vi "WriteRegisterArray.vi"(6 "Pause":u32, 7 "Mode":enum16{"Normal", "Config"}(ring), 8 "WriteSize":enum16{"1", "2", "4"}(ring), 9 "SclkDivider":u32=2, 10 "NumReg":i16, 11 "Register  Values":cluster{"Address":u8, "Value":u32}[](array[cluster])=[{"Address"=0, "Value"=0}, {"Address"=0, "Value"=0}, {"Address"=0, "Value"=0}, {"Address"=0, "Value"=0}, {"Address"=0, "Value"=0}, {"Address"=0, "Value"=0}, {"Address"=0, "Value"=0}, {"Address"=0, "Value"=0}, {"Address"=0, "Value"=0}, {"Address"=0, "Value"=0}, {"Address"=0, "Value"=0}, {"Address"=0, "Value"=0}, {"Address"=0, "Value"=0}, {"Address"=0, "Value"=0}, {"Address"=0, "Value"=0}, {"Address"=0, "Value"=0}, {"Address"=0, "Value"=0}, {"Address"=0, "Value"=0}, {"Address"=0, "Value"=0}, {"Address"=0, "Value"=0}]) -> ()   [LabVIEW 2012]
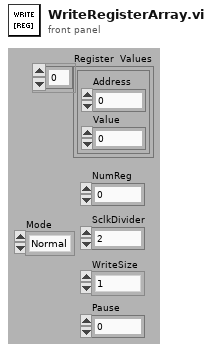
[diagram p1: front panel]
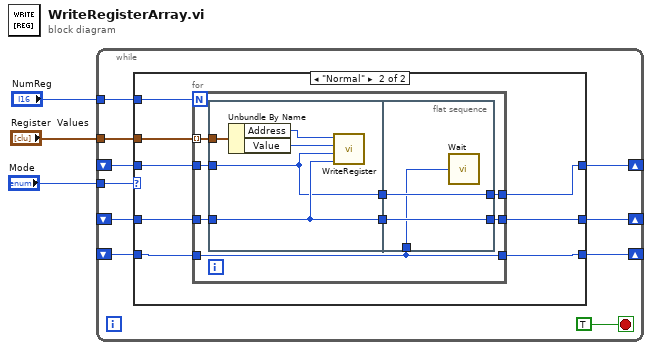
[diagram p0: block diagram]
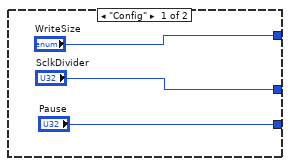
[diagram p2: hidden frame]
diagram:
  n1 = while {
    tunnel: "Register  Values" -> [w13]
    tunnel: "NumReg" -> [w12]
    tunnel: "Mode" -> [w10]
    shift-right: [w9] -> _
    shift-left: _ -> [w7]
    shift-right: [w8] -> _
    shift-left: _ -> [w6]
    shift-right: [w5] -> _
    shift-left: _ -> [w4]
    stop <- TRUE stop-if-true
    n2 = case shown="\"Normal\"" w10 {
      tunnel: w13 -> [_ w24]
      tunnel: w12 -> [_ w23]
      tunnel: ["WriteSize" w19] -> w9
      tunnel: ["SclkDivider" w20] -> w8
      tunnel: w7 -> [_ w22]
      tunnel: w6 -> [_ w21]
      tunnel: ["Pause" w17] -> w5
      tunnel: w4 -> [_ w18]
      frame "Config" {
      }
      frame "Normal" {
        n3 = for {
          N: w23 -> [_]
          tunnel: w24 -> [w32] mode=indexing
          tunnel: w22 -> [w31]
          tunnel: w21 -> [w30]
          tunnel: [w28] -> w20
          tunnel: [w27] -> w19
          tunnel: w18 -> [w25]
          tunnel: [w25] -> w17
          n4 = flat-sequence {
            tunnel: w32 -> [w37]
            tunnel: w31 -> [w33]
            tunnel: w30 -> [w34]
            tunnel: [w34] -> w29
            tunnel: [w33] -> w26
            tunnel: [w40] -> w28
            tunnel: w29 -> [w40]
            tunnel: [w39] -> w27
            tunnel: w26 -> [w39]
            tunnel: w25 -> [w38]
            frame #0 {
              n5 = Unbundle By Name(w37) -> ("Address"=w35:u8, "Value"=w36:u32)
              n6 = call "WriteRegister.vi"("Divider"=w34, "WriteSize"=w33, "RegisterValue"=w36, "RegisterAddress"=w35) -> ()  [unwired: 8 in]
            }
            frame #1 {
              n7 = call "Wait"("Count(Ticks)"=w38) -> ()  [unwired: 1 out]
            }
          }
        }
      }
    }
  }
